vi "练习 3.vi"() -> ()   [LabVIEW 2021]
panel:
  out "Waveform Graph":dynamicdata(graph)
  in  "stop":bool
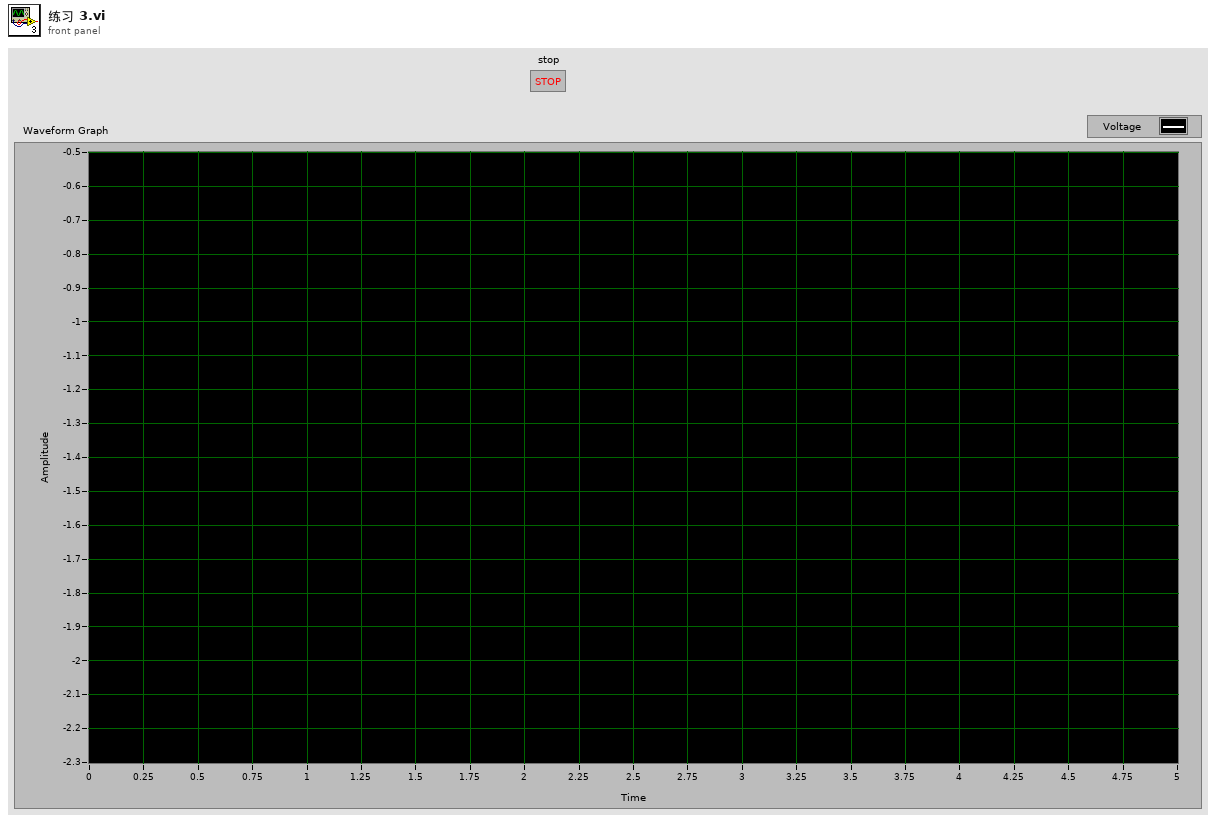
[diagram p1: front panel]
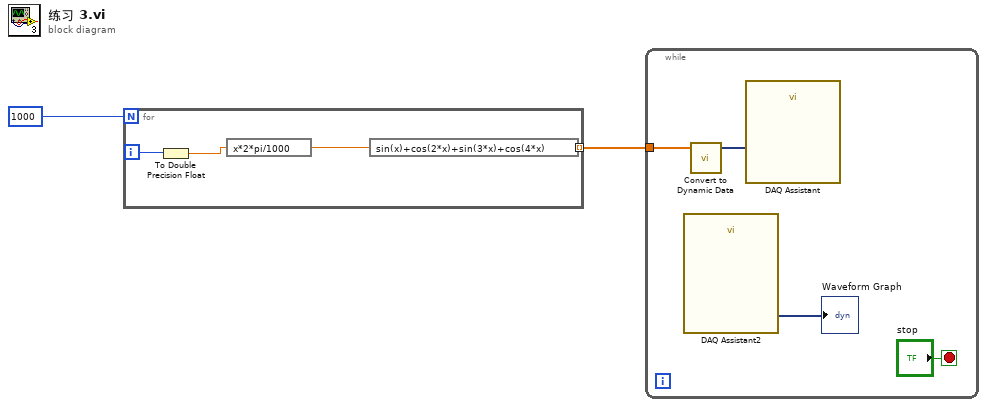
[diagram p0: block diagram]
diagram:
  n1 = for {
    N: 1000 -> [_]
    tunnel: [w5] -> w1 mode=indexing
    i -> [w4]
    n2 = To Double Precision Float(number=w4) -> (double precision float=w3:dbl)
    n3 = expression code="x*2*pi/1000"(w3) -> (w6:dbl)
    n4 = expression code="sin(x)+cos(2*x)+sin(3*x)+cos(4*x)"(w6) -> (w5:dbl)
  }
  n5 = while {
    tunnel: w1 -> [w10]
    stop <- "stop" stop-if-true
    n6 = call "DAQ Assistant2"() -> ("data"=→"Waveform Graph":dynamicdata)  [unwired: 17 in, 2 out]
    n7 = call "Convert to Dynamic Data"("Array"=w10) -> ("Dynamic Data Type"=w9:dynamicdata)  [unwired: 3 in]
    n8 = call "DAQ Assistant"("data"=w9) -> ()  [unwired: 16 in, 3 out]
  }
